vi "Generate Event.vi"(8 "error in (no error)":errorcluster, 10 "Event Data":refnum<class "Event.lvclass">, 11 "Event Sink in":refnum<class "Event Sink.lvclass">) -> (0 "error out":errorcluster, 3 "Event Sink out":refnum<class "Event Sink.lvclass">)   [LabVIEW 2016, in "Event Source.lvlib" / "Event Sink.lvclass"]
uses:
  Event Sink.lvclass
  C:/Program Files (x86)/National Instruments/LabVIEW 2016/vi.lib/ActorFramework/Actor/Actor.lvclass
  Event/Event.lvclass
  Event Sink.lvclass/Event Sink.ctl
  <vilib>/ActorFramework/Actor/Actor.lvclass/Actor.ctl
  <vilib>/ActorFramework/Message Enqueuer/Message Enqueuer.lvclass/Message Enqueuer.ctl
  properties/Read Event Source Enqueuer.vi
  properties/Read Paused.vi
  properties/Read Receive Only.vi
  <vilib>/ActorFramework/Message Enqueuer/Init from Existing Queue.vi
  <vilib>/ActorFramework/Message Enqueuer/Message Enqueuer.lvclass
  Event Source Messages/Receive and Broadcast Event Msg/Receive and Broadcast Event Msg.lvclass
  <vilib>/ActorFramework/Actor/Actor.lvclass
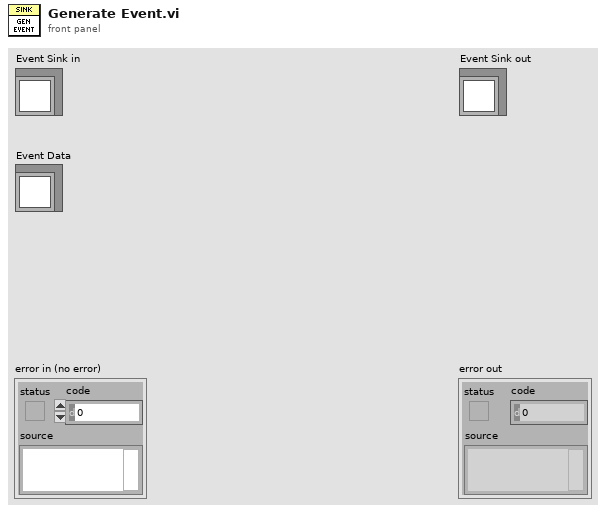
[diagram p1: front panel]
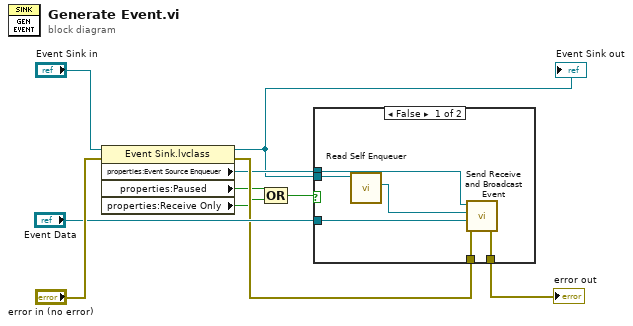
[diagram p0: block diagram]
diagram:
  n1 = property class="Event Sink.lvclass"(reference="Event Sink in", error in="error in (no error)") -> (reference out=w4:refnum<class "Event Sink.lvclass">, error out=w7:errorcluster, "properties:Event Source Enqueuer"=w5:refnum<class "Message Enqueuer.lvclass">, "properties:Paused"=w3:bool, "properties:Receive Only"=w2:bool)
  "Event Sink out" <- w4
  n2 = Compound Arithmetic op=OR(w3, w2) -> (w1:bool)
  n3 = case shown="False" w1 {
    tunnel: "Event Data" -> [w15 _]
    tunnel: w7 -> [w14 w17]
    tunnel: [w13 w17] -> w6
    tunnel: w5 -> [w12 _]
    tunnel: w4 -> [w11 _]
    frame False {
      n4 = call <vilib>:"Read Self Enqueuer.vi"("Actor"=w11) -> ("Self Enqueuer"=w16:refnum<class "Message Enqueuer.lvclass">)  [unwired: 10 in]
      n5 = call "Send Receive and Broadcast Event.vi"("error in (no error)"=w14, "Event Data"=w15, "Sink Enqueuer"=w16, "Message Enqueuer in"=w12) -> ("error out"=w13:errorcluster)  [unwired: 6 in, 1 out]
    }
    frame True {
    }
  }
  "error out" <- w6
